vi "PiezoClose.vi"(4 "error in (no error)":errorcluster, 7 "reference":refnum<k7>) -> (0 "error out":errorcluster, 3 "reference out":refnum<k7>)   [LabVIEW 2018]
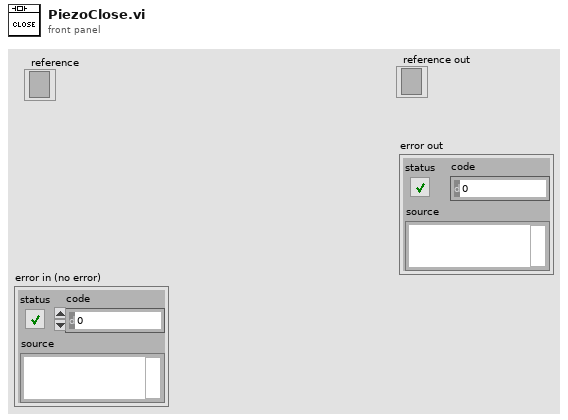
[diagram p1: front panel]
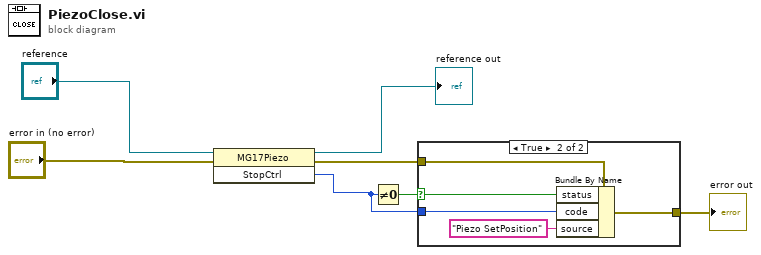
[diagram p0: block diagram]
diagram:
  n1 = invoke class="MG17Piezo" method="StopCtrl"(reference="reference", error in="error in (no error)") -> (reference out=→"reference out":refnum<k7>, error out=w3:errorcluster, "StopCtrl"=w1:i32)  [unwired: 1 in]
  n2 = Not Equal To 0?(x=w1) -> (x != 0?=w4:bool)
  n3 = case shown="True" w4 {
    selector: w4 -> [_ w12]
    tunnel: w3 -> [w8 w13]
    tunnel: [w8 w10] -> w2
    tunnel: w1 -> [_ w9]
    frame False {
    }
    frame True {
      n4 = Bundle By Name(cluster=w13, "status"=w12, "code"=w9, "source"="Piezo SetPosition") -> (w10:errorcluster)
    }
  }
  "error out" <- w2
